vi "Create.vi"() -> (3 "System Config Identity out":refnum<class "System Config Identity.lvclass">)   [LabVIEW 2020, in "Volatus.lvlib" / "System Config Identity.lvclass"]
uses:
  System Config Identity.lvclass
  System Config Identity.lvclass/System Config Identity.ctl
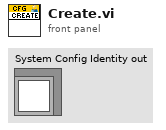
[diagram p1: front panel]
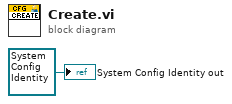
[diagram p0: block diagram]
diagram:
  "System Config Identity out" <- refnum<class "System Config Identity.lvclass"> refnum ("System Config Identity out")
